vi "MU Read Register I2C.vi"(7 "i2cSlaveAddress":u32, 8 "error in (no error)":errorcluster, 9 "registerCount":u32, 10 "registerAddress":u32, 11 "handle":u64) -> (0 "error out (no error)":errorcluster, 1 "registerCount out":u32, 2 "values":u32[](array[numeric]), 3 "function return":u32)   [LabVIEW 2017, in "MU_3SL_interface.lvlib"]
uses:
  MU_3SL_interface.lvlib
  lib/MU_3SL_interface.dll
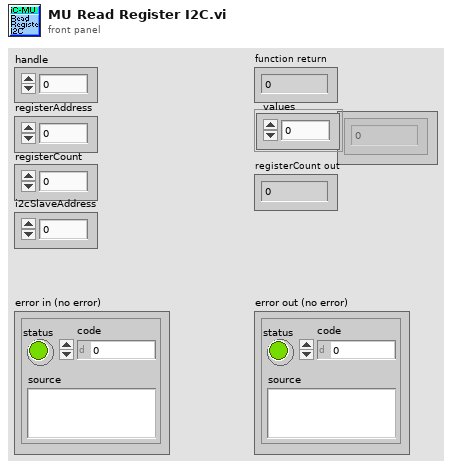
[diagram p1: front panel]
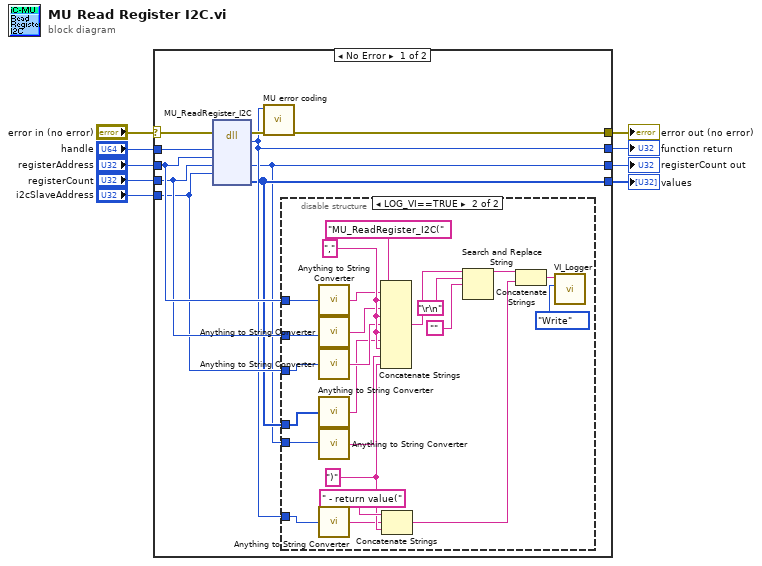
[diagram p0: block diagram]
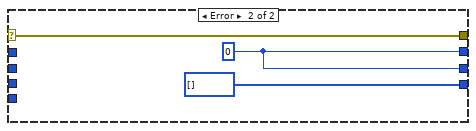
[diagram p3: hidden frame]
diagram:
  n1 = case shown="No Error" "error in (no error)" {
    selector: "error in (no error)" -> [w16 w45]
    tunnel: [w12 w43] -> w9
    tunnel: "handle" -> [w19 _]
    tunnel: [w17 w45] -> w7
    tunnel: "registerAddress" -> [w15 _]
    tunnel: "registerCount" -> [w14 _]
    tunnel: "i2cSlaveAddress" -> [w13 _]
    tunnel: [w11 u32[] [] ("pulData")] -> w2
    tunnel: [w10 w43] -> w1
    frame No Error {
      n2 = dll-call lib="C:/Users/bes/AppData/Roaming/work/mu_9so/icsubmodules/soft_mu_3sl_master/lv_interface/lib/MU_3SL_interface**.*" fn="MU_ReadRegister_I2C"(error in=w16, "handle"=w19, "registerAddress"=w15, "registerCount"=w14, "i2cSlaveAddress"=w13) -> (error out=w18:errorcluster, "return type"=w12:u32, "registerCount"=w10:u32, "values"=w11:u32[])  [unwired: 6 in, 1 out]
      n3 = call "MU error coding.vi"("error in (no error)"=w18, "function return in"=w12) -> ("error out"=w17:errorcluster)  [unwired: 9 in]
      n4 = disable-structure shown="LOG_VI==TRUE" {
        disable-tunnel: w12 -> [_ w21]
        disable-tunnel: w15 -> [_ w31]
        disable-tunnel: w14 -> [_ w29]
        disable-tunnel: w13 -> [_ w27]
        disable-tunnel: w11 -> [_ w25]
        disable-tunnel: w10 -> [_ w23]
        frame condition #0 {
        }
        frame condition #1 (active) {
          w36 = ")" ("string")
          w37 = "," ("string")
          n5 = call "Anything to String Converter.vi"("anything"=w31) -> ("String"=w30:string)
          n6 = call "Anything to String Converter.vi"("anything"=w29) -> ("String"=w28:string)
          n7 = call "Anything to String Converter.vi"("anything"=w27) -> ("String"=w26:string)
          n8 = call "Anything to String Converter.vi"("anything"=w25) -> ("String"=w24:string)
          n9 = call "Anything to String Converter.vi"("anything"=w23) -> ("String"=w22:string)
          n10 = call "Anything to String Converter.vi"("anything"=w21) -> ("String"=w20:string)
          n11 = Concatenate Strings("MU_ReadRegister_I2C(" ("Info in"), w30, w37, w28, w37, w26, w37, w24, w37, w22, w36) -> (w32:string)
          n12 = Concatenate Strings(" - return value(" ("string"), w20, w36) -> (w40:string)
          n13 = Search and Replace String(input string=w32, search string="\r\n", replace string="") -> (result string=w33:string)  [unwired: 5 in, 3 out]
          n14 = Concatenate Strings(w33, w40) -> (w39:string)
          n15 = call "VI_Logger.vi"("Action (Read)"=enum16{"Write", "Read"}."Write", "Info in"=w39) -> ()  [unwired: 8 in, 2 out]
        }
      }
    }
    frame Error {
      w43 = u32 0
    }
  }
  "function return" <- w9
  "error out (no error)" <- w7
  "values" <- w2
  "registerCount out" <- w1
